vi "Read value.vi"(8 "error in (no error)":errorcluster, 11 "JSON String in":refnum<class "JSON Null.lvclass">=refnum) -> (0 "error out":errorcluster, 2 "value":bool, 3 "JSON String out":refnum<class "JSON Null.lvclass">)   [LabVIEW 2017]
uses:
  JSON Null.lvclass
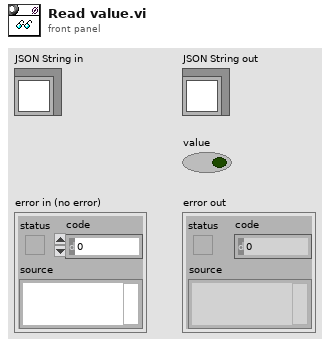
[diagram p1: front panel]
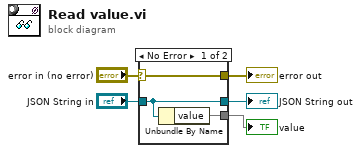
[diagram p0: block diagram]
diagram:
  n1 = case shown="No Error" "error in (no error)" {
    selector: "error in (no error)" -> [w8 w9]
    tunnel: [w8 w9] -> w4
    tunnel: [w7 w10] -> w2
    tunnel: "JSON String in" -> [w7 w10]
    tunnel: [w6 _] -> w1
    frame No Error {
      n2 = Unbundle By Name(w7) -> ("value"=w6)
    }
    frame Error {
    }
  }
  "error out" <- w4
  "JSON String out" <- w2
  "value" <- w1
